vi "Convert Error to MCL ItemName.vi"(1 "Error To Display":T1) -> (0 "ItemName":string[](array[string]))   [LabVIEW 2023, in "Error Manager.lvlib"]
doc: "Blank VI with error handling."
uses:
  Error Manager.lvlib
  Handled Error (cluster).ctl
  Read-Unread Status (enum).ctl
panel:
  # "Input\nInputs to the VI"
  # "Development\nControls or indicators that are useful for development or testing, but which are not outputs of the VI."
  # "Output\nOutputs of the VI"
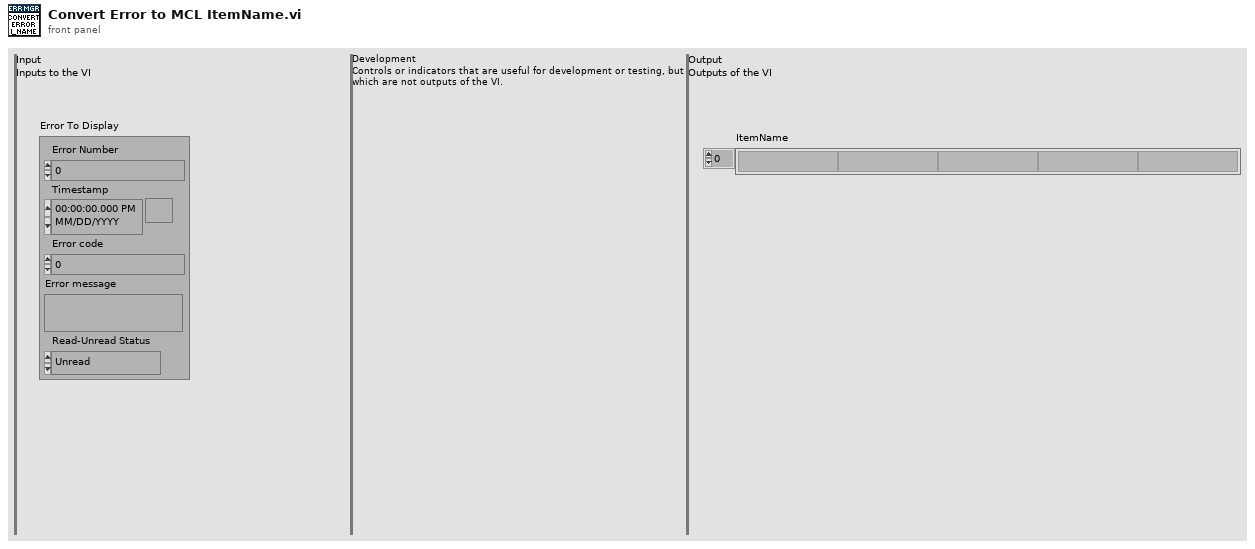
[diagram p1: front panel]
types:
  T1 = typedef "Error Manager.lvlib/Handled Error (cluster).ctl" = cluster{"Error Number":i32, "Timestamp":timestamp, "Error code":i32, "Error message":string, "Read-Unread Status":T2}
  T2 = typedef "Error Manager.lvlib/Read-Unread Status (enum).ctl" = enum16{"Unread", "Read"}
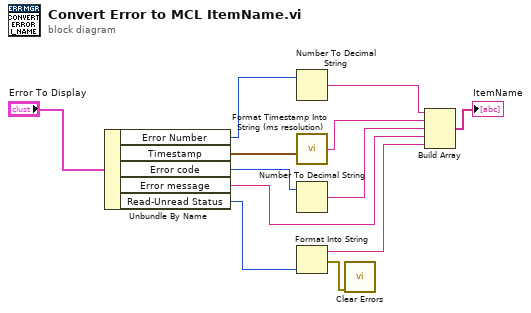
[diagram p0: block diagram]
diagram:
  n1 = Unbundle By Name("Error To Display") -> ("Error Number"=w3:i32, "Timestamp"=w2:timestamp, "Error code"=w11:i32, "Error message"=w9:string, "Read-Unread Status"=w8:T2)
  n2 = Number To Decimal String(number=w3) -> (decimal integer string=w4:string)  [unwired: 1 in]
  n3 = call "Format Timestamp Into String (ms resolution).vi"("Timestamp"=w2) -> ("Timestamp String (ms resolution)"=w1:string)
  n4 = Number To Decimal String(number=w11) -> (decimal integer string=w10:string)  [unwired: 1 in]
  n5 = Format Into String(w8) -> (resulting string=w7:string, error out=w6:errorcluster)  [unwired: 3 in]
  n6 = call <vilib>:"Clear Errors.vi"("error in (no error)"=w6) -> ()  [unwired: 5 in, 2 out]
  n7 = Build Array(w4, w1, w10, w9, w7) -> (→"ItemName":string[])
